vi "SCRIPT_LOAD.vi"(0 "TCP session in":refnum<k5>, 5 "lua script":string, 11 "error in":errorcluster) -> (4 "TCP session out":refnum<k5>, 6 "Data":T1, 8 "script SHA1":string, 15 "error out":errorcluster)   [LabVIEW 2023]
uses:
  SubVIs/Controls/redis-data.ctl
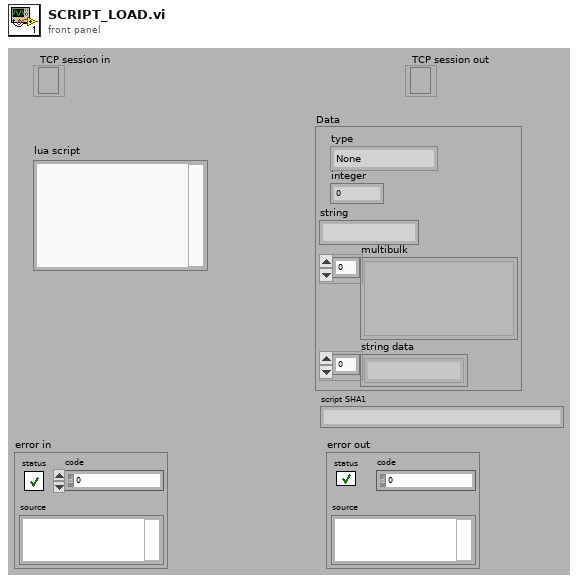
[diagram p1: front panel]
types:
  T1 = typedef "redis-data.ctl" = cluster{"type":enum16{"None", "Error", "Status", "Nil", "Integer", "String", "Multibulk"}, "integer":i64, "string":string, "multibulk":variant[], "string data":string[]}
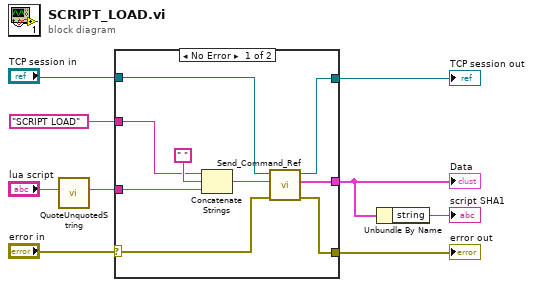
[diagram p0: block diagram]
diagram:
  n1 = call "QuoteUnquotedString.vi"("String in"="lua script") -> ("String out"=w1:string)  [unwired: 10 in]
  n2 = case shown="No Error" "error in" {
    selector: "error in" -> [w15 w20]
    tunnel: w1 -> [w12 _]
    tunnel: "SCRIPT LOAD" -> [w17 _]
    tunnel: "TCP session in" -> [w11 w19]
    tunnel: [w14 w20] -> w7
    tunnel: [w13 _] -> w3
    tunnel: [w10 w19] -> w4
    frame No Error {
      n3 = Concatenate Strings(w17, " ", w12) -> (w16:string)
      n4 = call "Send_Command_Ref.vi"("error in"=w15, "command"=w16, "TCP session in"=w11) -> ("error out"=w14:errorcluster, "Data"=w13:T1, "TCP session out"=w10:refnum<k5>)  [unwired: 6 in]
    }
    frame Error {
    }
  }
  "error out" <- w7
  "TCP session out" <- w4
  "Data" <- w3
  n5 = Unbundle By Name(w3) -> ("string"=→"script SHA1":string)
